vi "YokoGS200 Get Level.vi"(0 "VISA Rsrc":refnum<visa-resource-name>="SR530", 3 "error in (no error)":errorcluster) -> (7 "VISA Rsrc Out":refnum<visa-resource-name>="GPIB0::12::INSTR", 8 "Output Level":dbl, 10 "error out":errorcluster)   [LabVIEW 2019]
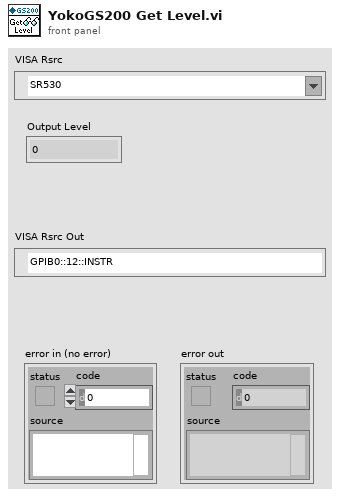
[diagram p1: front panel]
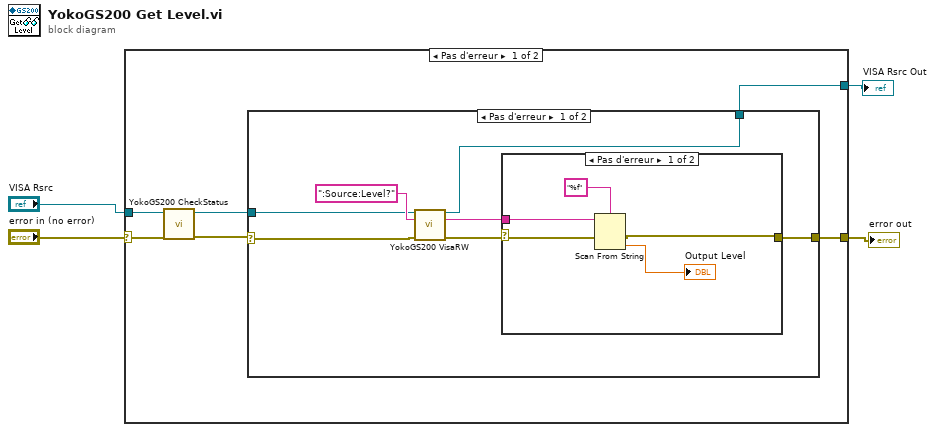
[diagram p0: block diagram]
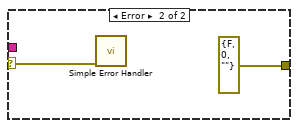
[diagram p2: hidden frame]
diagram:
  n1 = case shown="Pas d'erreur" "error in (no error)" {
    selector: "error in (no error)" -> [w9 w27]
    tunnel: "VISA Rsrc" -> [w8 w28]
    tunnel: [w10 w27] -> w2
    tunnel: [w5 w28] -> w1
    frame No Error {
      n2 = call <userlib>:"YokoGS200 CheckStatus.vi"("error in (no error)"=w9, "VISA Rsrc"=w8) -> ("error out"=w7:errorcluster, "VISA Rsrc Out"=w6:refnum<visa-resource-name>)  [unwired: 6 in, 2 out]
      n3 = case shown="Pas d'erreur" w7 {
        selector: w7 -> [w13 w26]
        tunnel: [w16 w26] -> w10
        tunnel: w6 -> [w12 w25]
        tunnel: [w11 w25] -> w5
        frame No Error {
          n4 = call <userlib>:"YokoGS200 VisaRW.vi"("VISA Rsrc"=w12, "ChaineCom"=":Source:Level?" ("initial string"), "error in (no error)"=w13) -> ("VISA Rsrc Out"=w11:refnum<visa-resource-name>, "ChaineRep"=w14:string, "error out"=w15:errorcluster)  [unwired: 8 in, 2 out]
          n5 = case shown="Pas d'erreur" w15 {
            selector: w15 -> [w22 w23]
            tunnel: [w19 errorcluster {"status"=FALSE, "code"=0, "source"=""} ("error IO")] -> w16
            tunnel: w14 -> [w21 _]
            frame No Error {
              n6 = Scan From String(format string="%f", input string=w21, error in=w22) -> (error out=w19:errorcluster, output 1=→"Output Level":dbl)  [unwired: 2 in, 2 out]
            }
            frame Error {
              n7 = call <vilib>:"Simple Error Handler.vi"("error in (no error)"=w23) -> ()  [unwired: 4 in, 5 out]
            }
          }
        }
        frame Error {
        }
      }
    }
    frame Error {
    }
  }
  "error out" <- w2
  "VISA Rsrc Out" <- w1
